vi "Calculate Voltage Magnitude Measurements.vi"(9 "Voltage Waveform":dbl[](array[numeric]), 10 "Event.Parameters":T1={"Shots"=0, "Shot.InitialVoltage"=0.0, "Shot.Stages"=0, "Stages"=[{"Stage.Dwell.Level"=0.0, "PullIn.Type"=enum."Pull In Transition Dwells", "PullIn.Level"=0.0, "Transition.Type"=enum."Stage Transition Voltage Level", "Transition.Level"=0.0}]}, 11 "Shot Info Array":T5[](array[typedef]) {"Results"."Off-Stage Avg Current" format="%#.6g"; "Results"."Total Voltage Pulses" format="%#.6g"; "Results"."Off-Stage Min Current" format="%#.6g"; "Results"."Off-Stage Max Current" format="%#.6g"}) -> (3 "Shot Info Array":T5[](array[typedef]) {"Results"."Off-Stage Avg Current" format="%#.6g"; "Results"."Total Voltage Pulses" format="%#.6g"; "Results"."Off-Stage Min Current" format="%#.6g"; "Results"."Off-Stage Max Current" format="%#.6g"})   [LabVIEW 2015, in "Fuel Injector Analysis Addon Engine.lvlib"]
uses:
  Fuel Injector Analysis Addon Engine.lvlib
  Controls/Shot Information Control.ctl
  Types/Stage.Measurements.ctl
  Shared/Types/Shot.Parameters.ctl
  Shared/Types/Stage.Parameters.ctl
  Shared/Types/Stage.PullIn.Types.ctl
  Shared/Types/Stage.Transition.Types.ctl
  <vilib>/Analysis/baseanly.llb/Mean.vi
  <vilib>/Analysis/baseanly.llb/Mean (DBL).vi
  Shared/Constants.vi
  Shared/Fuel Injector Analysis Addon Shared.lvlib
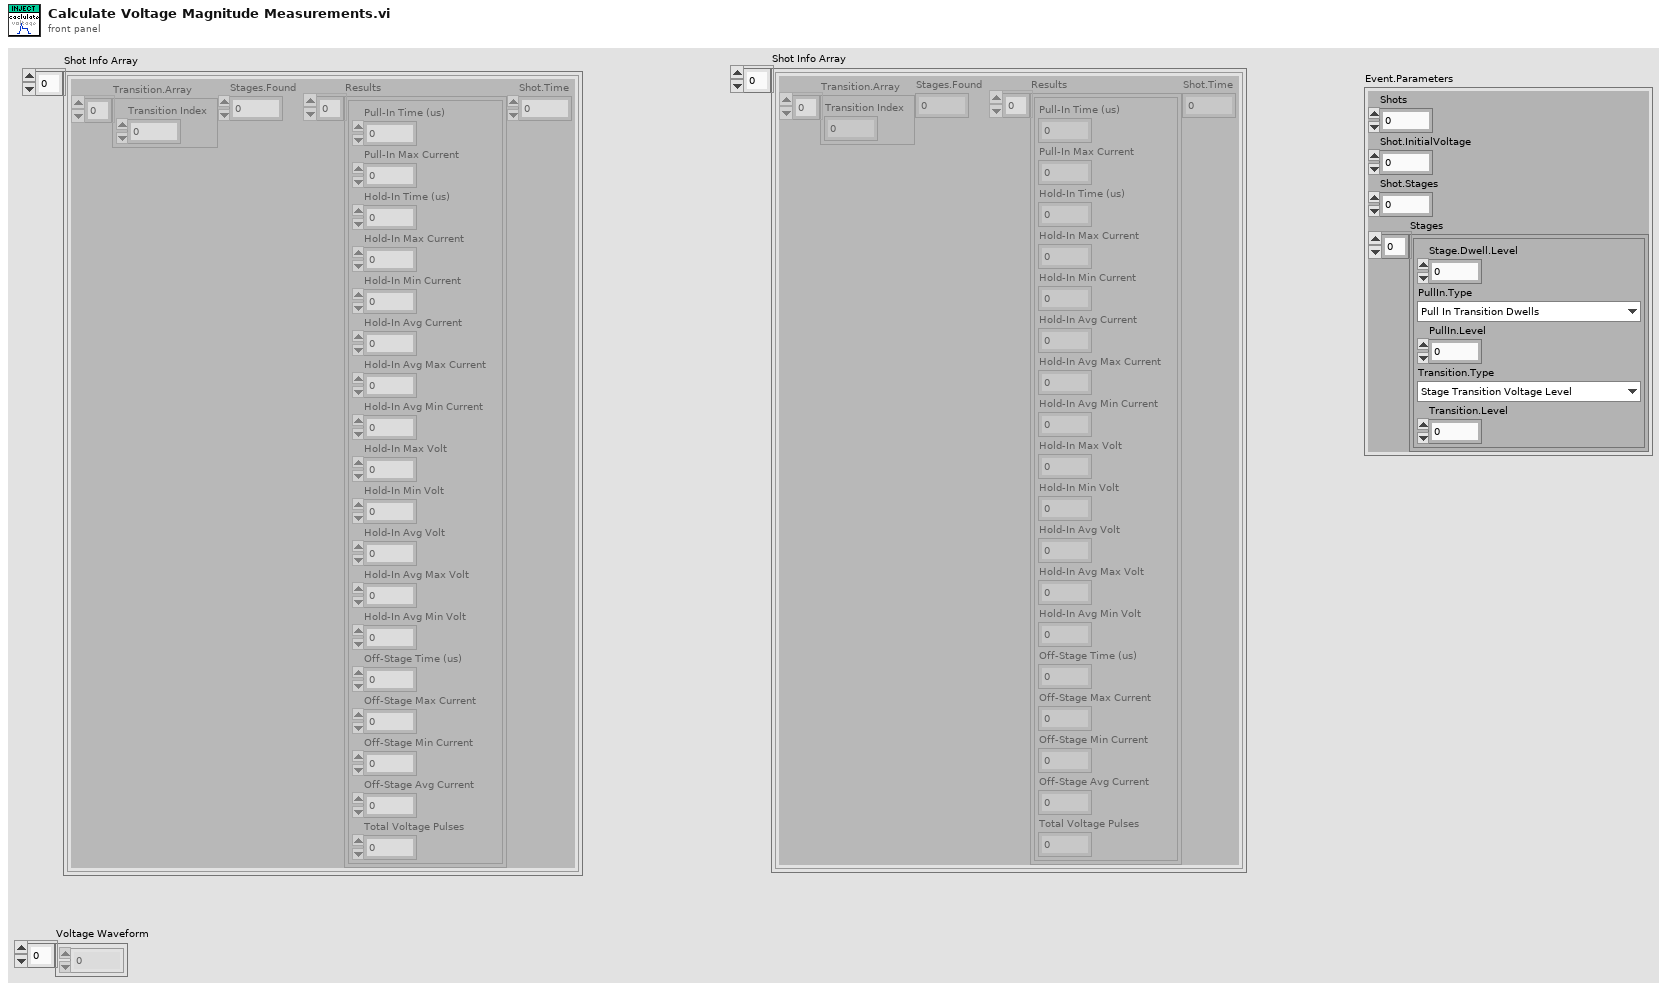
[diagram p1: front panel]
types:
  T1 = typedef "Fuel Injector Analysis Addon Shared.lvlib/Shot.Parameters.ctl" = cluster{"Shots":u32, "Shot.InitialVoltage":dbl, "Shot.Stages":u32, "Stages":T2[]}
  T2 = typedef "Fuel Injector Analysis Addon Shared.lvlib/Stage.Parameters.ctl" = cluster{"Stage.Dwell.Level":dbl, "PullIn.Type":T3, "PullIn.Level":dbl, "Transition.Type":T4, "Transition.Level":dbl}
  T3 = typedef "Fuel Injector Analysis Addon Shared.lvlib/Stage.PullIn.Types.ctl" = enum8{"Pull In Transition Dwells", "Pull In Transition Current Drop"}
  T4 = typedef "Fuel Injector Analysis Addon Shared.lvlib/Stage.Transition.Types.ctl" = enum8{"Stage Transition Dwell Time", "Stage Transition Voltage Level", "Stage Transition Current Drop"}
  T5 = typedef "Fuel Injector Analysis Addon Engine.lvlib/Shot Information Control.ctl" = cluster{"Transition.Array":i32[], "Stages.Found":u16, "Results":T6[], "Shot.Time":dbl}
  T6 = typedef "Fuel Injector Analysis Addon Engine.lvlib/Stage.Measurements.ctl" = cluster{"Pull-In Time (us)":dbl, "Pull-In Max Current":dbl, "Hold-In Time (us)":dbl, "Hold-In Max Current":dbl, "Hold-In Min Current":dbl, "Hold-In Avg Current":dbl, "Hold-In Avg Max Current":dbl, "Hold-In Avg Min Current":dbl, "Hold-In Max Volt":dbl, "Hold-In Min Volt":dbl, "Hold-In Avg Volt":dbl, "Hold-In Avg Max Volt":dbl, "Hold-In Avg Min Volt":dbl, "Off-Stage Time (us)":dbl, "Off-Stage Max Current":dbl, "Off-Stage Min Current":dbl, "Off-Stage Avg Current":dbl, "Total Voltage Pulses":dbl}
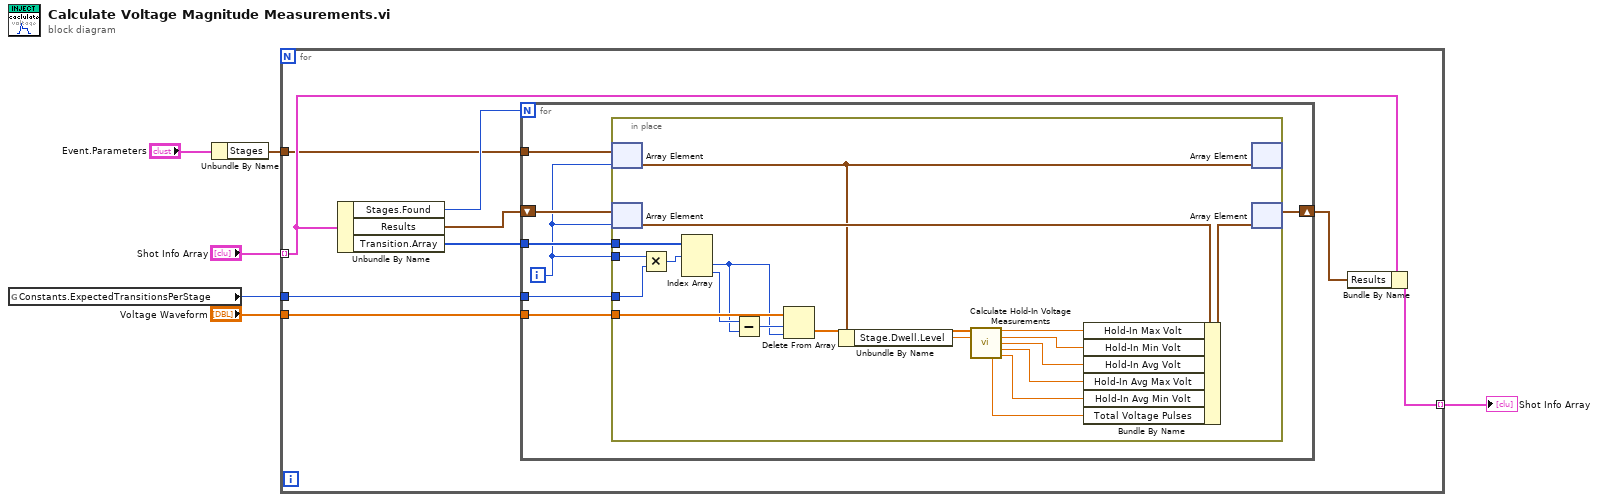
[diagram p0: block diagram]
diagram:
  n1 = global read "Constants.vi" "Constants.ExpectedTransitionsPerStage"() -> (w3:u32)
  n2 = Unbundle By Name("Event.Parameters") -> ("Stages"=w1:T2[])
  n3 = for {
    tunnel: "Voltage Waveform" -> [w14]
    tunnel: "Shot Info Array" -> [w12] mode=indexing
    tunnel: [w15] -> w6 mode=indexing
    tunnel: w3 -> [w8]
    tunnel: w1 -> [w7]
    n4 = Unbundle By Name(w12) -> ("Stages.Found"=w10:u16, "Results"=w11:T6[], "Transition.Array"=w13:i32[])
    n5 = for {
      N: w10 -> [_]
      tunnel: w14 -> [w22]
      tunnel: w13 -> [w21]
      shift-right: [w19] -> w9
      shift-left: w11 -> [w20]
      tunnel: w8 -> [w18]
      tunnel: w7 -> [w17]
      i -> [w16]
      n6 = in-place {
        in-place-border: w22 -> [w41]
        in-place-border: w21 -> [w40]
        in-place-border: w16 -> [w37]
        in-place-border: w18 -> [w35]
        n7 = in-place-array #1(w17, w16) -> (w24:T2)
        n8 = in-place-array #2(w20, w16) -> (w39:T6)
        n9 = Multiply(x=w37, y=w35) -> (x*y=w36:u32)
        n10 = Index Array(array=w40, index #1=w36) -> (element #2=w23:i32, element #3=w34:i32)  [unwired: 2 in, 1 out]
        n11 = Subtract(x=w34, y=w23) -> (x-y=w33:i32)
        n12 = Delete From Array(array=w41, length=w33, index=w23) -> (deleted portion=w26:dbl[])  [unwired: 1 out]
        n13 = Unbundle By Name(w24) -> ("Stage.Dwell.Level"=w25:dbl)
        n14 = call "Calculate Hold-In Voltage Measurements.vi"("Stage Voltage Section"=w26, "Stage.Dwell.Level"=w25) -> ("Max Stage"=w32:dbl, "Min Stage"=w31:dbl, "Avg Stage"=w30:dbl, "Avg Max Stage"=w29:dbl, "# of Pulses"=w27:dbl, "Avg Min Stage"=w28:dbl)  [unwired: 8 in]
        n15 = Bundle By Name(cluster=w39, "Hold-In Max Volt"=w32, "Hold-In Min Volt"=w31, "Hold-In Avg Volt"=w30, "Hold-In Avg Max Volt"=w29, "Hold-In Avg Min Volt"=w28, "Total Voltage Pulses"=w27) -> (w38:T6)
        n16 = in-place-array #1(w24) -> ()  [unwired: 2 out]
        n17 = in-place-array #2(w38) -> (w19:T6[])  [unwired: 1 out]
      }
    }
    n18 = Bundle By Name(cluster=w12, "Results"=w9) -> (w15:T5)
  }
  "Shot Info Array" <- w6
